vi "GetBARPressure.vi"(1 "BAR ID Number":i32) -> (0 "Pressure":dbl)   [LabVIEW 2011]
uses:
  GlobalVariables.vi
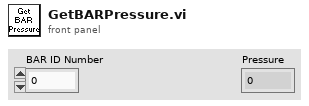
[diagram p1: front panel]
types:
  T1 = typedef "BAR Cluster.ctl" = cluster{"Pressure":dbl}
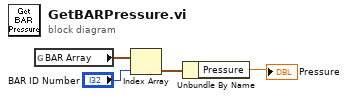
[diagram p0: block diagram]
diagram:
  n1 = global read "GlobalVariables.vi" "BAR Array"() -> (w4:T1[])
  n2 = Index Array(array=w4, index="BAR ID Number") -> (element=w2:T1)
  n3 = Unbundle By Name(w2) -> ("Pressure"=→"Pressure":dbl)
